vi "Set Voltage Output.vi"(8 "error in (no error)":errorcluster, 10 "Voltage Output":refnum<class "Voltage Output.lvclass">, 11 "Ramp Voltage In":refnum<class "Ramp Voltage.lvclass">) -> (0 "error out":errorcluster, 3 "Ramp Voltage Out":refnum<class "Ramp Voltage.lvclass">)   [LabVIEW 2020, in "High Level PSU With Tests.lvlib" / "Ramp Voltage.lvclass"]
uses:
  Ramp Voltage.lvclass
  Voltage Output/Voltage Output.lvclass
  Ramp Voltage.lvclass/Ramp Voltage.ctl
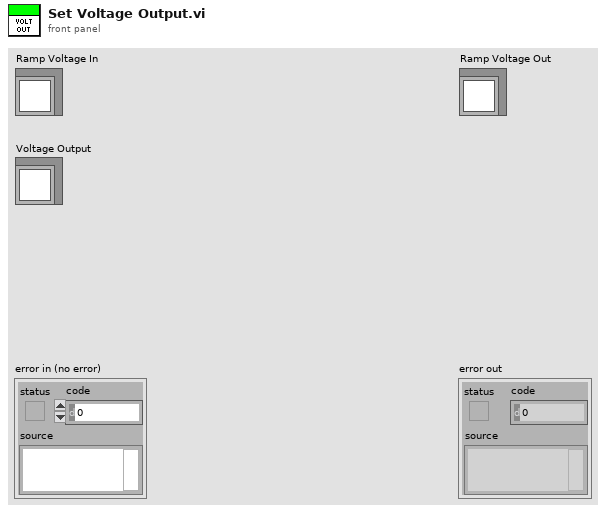
[diagram p1: front panel]
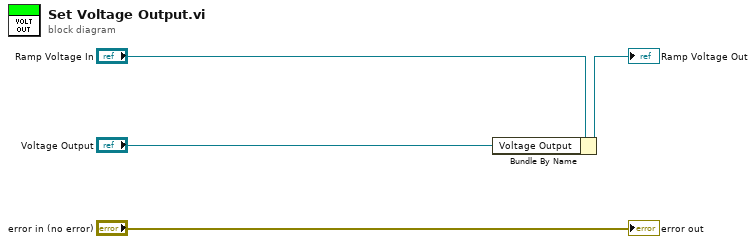
[diagram p0: block diagram]
diagram:
  n1 = Bundle By Name(cluster="Ramp Voltage In", "Voltage Output"="Voltage Output") -> (→"Ramp Voltage Out":refnum<class "Ramp Voltage.lvclass">)
  "error out" <- "error in (no error)"
